vi "Set Error Constant Value.vi"(8 "error in (no error)":errorcluster, 10 "error":errorcluster, 11 "VI in":refnum<vi>) -> (0 "error out":errorcluster, 3 "VI out":refnum<vi>)   [LabVIEW 2016]
uses:
  <vilib>/Utility/traverseref.llb/TRef TravTarget.ctl
  <vilib>/Utility/traverseref.llb/VI Scripting - Traverse.lvlib
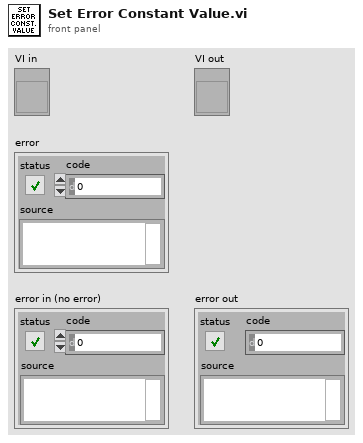
[diagram p1: front panel]
types:
  T1 = typedef "TRef TravTarget.ctl" = enum16{"FP", "BD", "Other"}
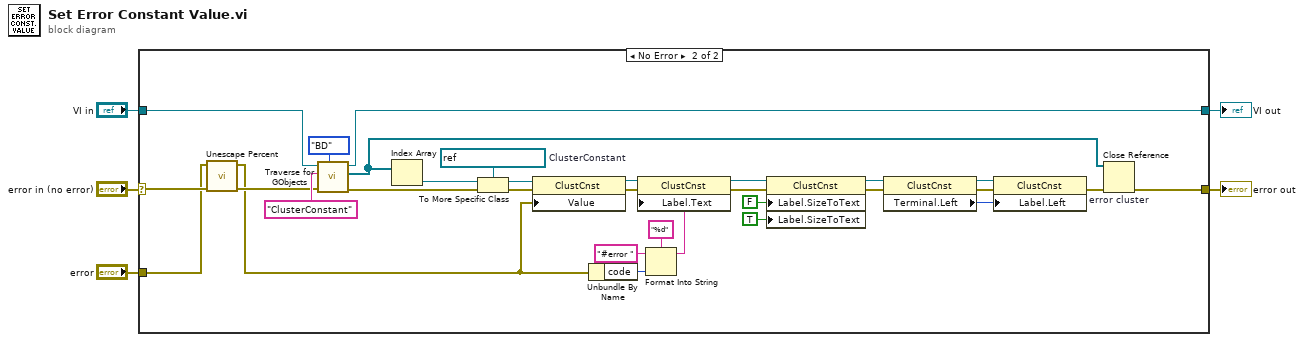
[diagram p0: block diagram]
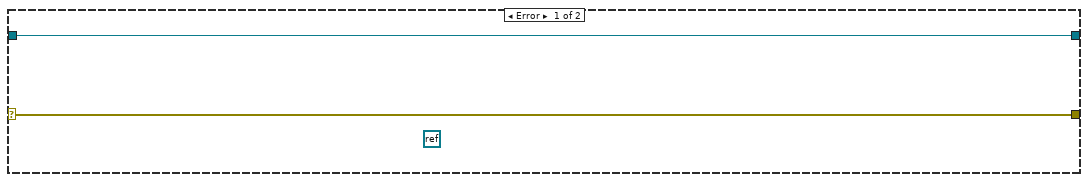
[diagram p2: hidden frame]
diagram:
  n1 = case shown="No Error" "error in (no error)" {
    selector: "error in (no error)" -> [w7 w11]
    tunnel: [w6 w29] -> w5
    tunnel: "VI in" -> [w6 w37]
    tunnel: [w7 w21] -> w2
    tunnel: "error" -> [_ w8]
    frame Error {
      (unwired) refnum<k0> refnum
    }
    frame No Error {
      w34 = refnum<vi> refnum  # ClusterConstant
      n2 = call "Unescape Percent.vi"("error in (no error)"=w11, "new error in"=w8) -> ("error out"=w10:errorcluster, "new error out"=w9:errorcluster)  [unwired: 8 in]
      n3 = call <vilib>:"Traverse for GObjects.vi"("Traverse Target"=TRef_TravTarget."BD", "error in (no error)"=w10, "Class Name"="ClusterConstant", "VI Refnum"=w37) -> ("error out"=w35:errorcluster, "References"=w23:refnum<vi>[], "dup VI Refnum"=w29:refnum<vi>)  [unwired: 4 in, 1 out]
      n4 = Index Array(array=w23) -> (element=w28:refnum<vi>)  [unwired: 1 in]
      n5 = To More Specific Class(target class=w34, reference=w28, error in=w35) -> (specific class reference=w36:refnum<vi>, error out=w38:errorcluster)
      n6 = property class="ClustCnst"(reference=w36, error in=w38, "Value"=w9) -> (reference out=w31:refnum<vi>, error out=w30:errorcluster)
      n7 = Unbundle By Name(w9) -> ("code"=w19:i32)
      n8 = Format Into String(format string="%d", initial string="#error " ("format string"), w19) -> (resulting string=w17:string)  [unwired: 1 in, 1 out]
      n9 = property class="ClustCnst"(reference=w31, error in=w30, "Label.Text"=w17) -> (reference out=w15:refnum<vi>, error out=w27:errorcluster)
      n10 = property class="ClustCnst"(reference=w15, error in=w27, "Label.SizeToText"=FALSE ("Label.Size to Text?"), "Label.SizeToText"=TRUE ("Label.Size to Text?")) -> (reference out=w14:refnum<vi>, error out=w16:errorcluster)
      n11 = property class="ClustCnst"(reference=w14, error in=w16) -> (reference out=w26:refnum<vi>, error out=w24:errorcluster, "Terminal.Left"=w25:i32)
      n12 = property class="ClustCnst"(reference=w26, error in=w24, "Label.Left"=w25) -> (error out=w22:errorcluster)  [unwired: 1 out]
      n13 = Close Reference "error cluster"(reference=w23, error in (no error)=w22) -> (error out=w21:errorcluster)
    }
  }
  "VI out" <- w5
  "error out" <- w2
